vi "Read All Errors.vi"(8 "error in (no error)":errorcluster, 11 "Item Ref in":T2 format="%.0x") -> (0 "error out":errorcluster, 1 "VeriStand Errors":T1[](array[typedef]), 2 "Keys":string[](array[string]), 3 "Item Ref out":T2 format="%.0x")   [LabVIEW 2027, in "VeriStand Error API.lvlib"]
doc: "<B>Read All Errors</B> returns an array of <B>Keys</B> and an array of error clusters for all of the errors thrown be the item referenced."
uses:
  VeriStand Error API.lvlib
  <vilib>/NI VeriStand/Custom Device API/Custom Device API.lvlib
  C:/NetCore/niveristand-custom-device-development-tools/error-api/Source/Read All Errors.vi/NationalInstruments.VeriStand.SystemStorage
  NationalInstruments.VeriStand.SystemStorage
  VeriStand Error.ctl
  <vilib>/NI VeriStand/Custom Device API/Custom Device Item Ref.ctl
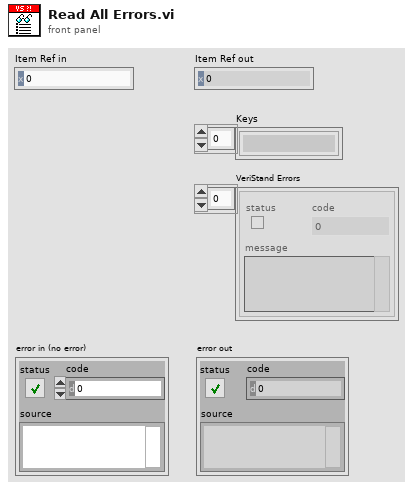
[diagram p1: front panel]
types:
  T1 = typedef "VeriStand Error API.lvlib/VeriStand Error.ctl" = cluster{"status":bool, "code":i32, "message":string}
  T2 = typedef "Custom Device API.lvlib/Custom Device Item Ref.ctl" = u64
  T3 = typedef "Custom Device API.lvlib/Custom Device Pointer.ctl" = refnum<k24>
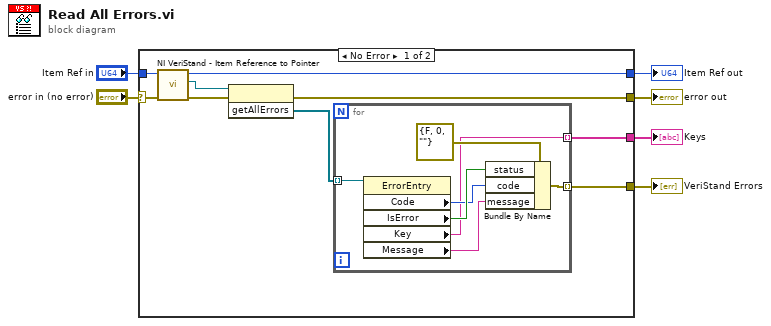
[diagram p0: block diagram]
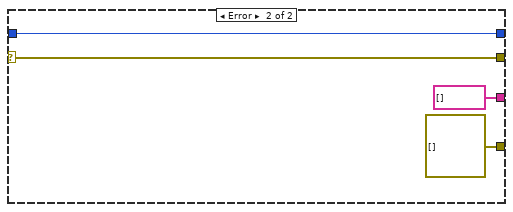
[diagram p2: hidden frame]
diagram:
  n1 = case shown="No Error" "error in (no error)" {
    selector: "error in (no error)" -> [w14 w26]
    tunnel: "Item Ref in" -> [w15 w25]
    tunnel: [w12 w25] -> w4
    tunnel: [w10 w26] -> w3
    tunnel: [w8 string[] []] -> w2
    tunnel: [w7 T1[] []] -> w1
    frame No Error {
      n2 = call <vilib>:"NI VeriStand - Item Reference to Pointer.vi"("error in (no error)"=w14, "Item Ref in"=w15) -> ("error out"=w11:errorcluster, "Node Pointer"=w13:T3, "Item Ref out"=w12:T2)  [unwired: 6 in, 1 out]
      n3 = invoke method="getAllErrors"(reference=w13, error in=w11) -> (error out=w10:errorcluster, "getAllErrors"=w9:refnum<k39>[])  [unwired: 1 in, 1 out]
      n4 = for {
        tunnel: w9 -> [w22] mode=indexing
        tunnel: [w17] -> w8 mode=indexing
        tunnel: [w16] -> w7 mode=indexing
        n5 = property class="ErrorEntry"(reference=w22) -> ("Code"=w19:i32, "IsError"=w20:bool, "Key"=w17:string, "Message"=w18:string)  [unwired: 1 in, 2 out]
        n6 = Bundle By Name(cluster=T1 {"status"=FALSE, "code"=0, "message"=""} ("VeriStand Error In"), "status"=w20, "code"=w19, "message"=w18) -> (w16:T1)
      }
    }
    frame Error {
    }
  }
  "error out" <- w3
  "Item Ref out" <- w4
  "Keys" <- w2
  "VeriStand Errors" <- w1
